vi "Example.vi"() -> ()   [LabVIEW 2014, in "TE Cooler.lvlib"]
uses:
  TE Cooler.lvlib
  <userlib>/_Session Fwk/Session - Root.lvclass
  reusable/Session APIs/File Access/Config Data/Config Data.lvclass
  reusable/Session APIs/File Access/Config Data/Config Session.ctl
  reusable/Session APIs/Session Log/System Log.lvclass
  TE Cooler.lvclass
  Data/TECData.lvclass
panel:
  out "error out":errorcluster
  out "Power":sgl
  in  "STOP":bool
  out "Input 1":sgl(graph)
  out "Input 2":sgl(graph)
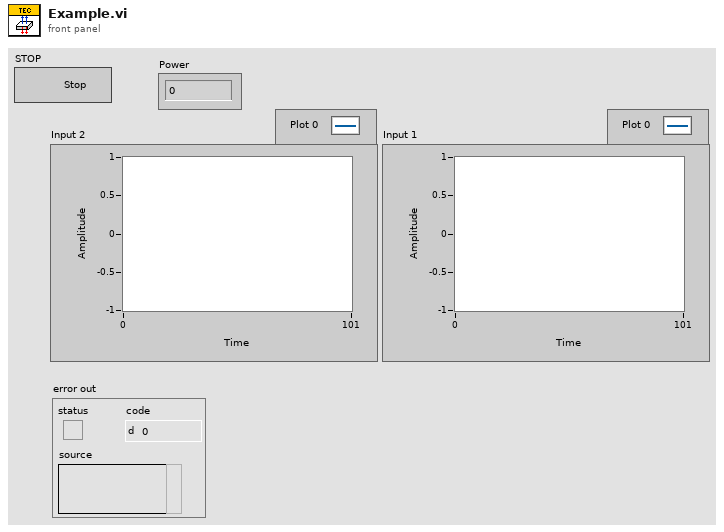
[diagram p1: front panel]
types:
  T1 = typedef "Config Data.lvclass/Config Session.ctl" = refnum<data-value>
  T2 = typedef "Session - Root.lvclass/Session Handle.ctl" = refnum<data-value>
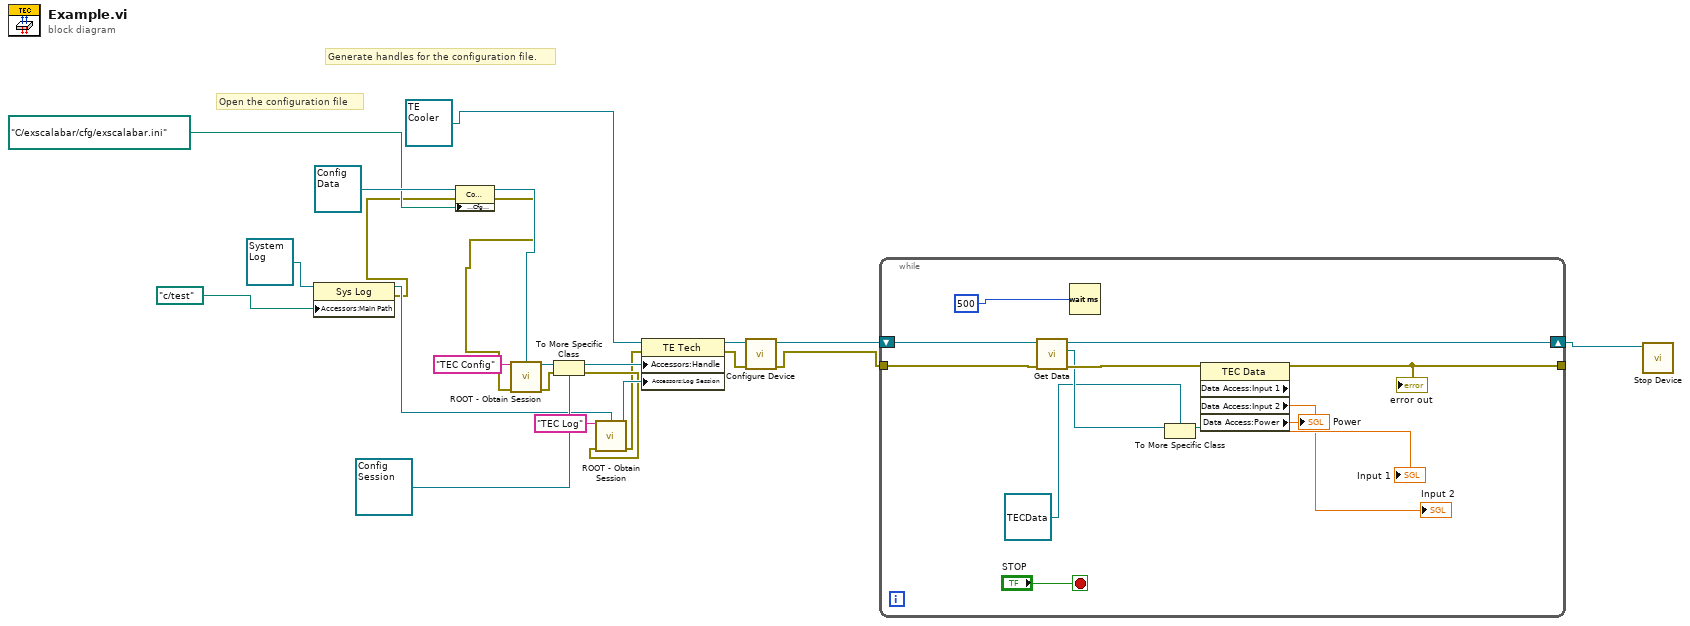
[diagram p0: block diagram]
diagram:
  # "Open the configuration file"
  # "Generate handles for the configuration file."
  n1 = property class="Sys Log"(reference=refnum<class "System Log.lvclass"> refnum ("Sys Log"), "Accessors:Main Path"=path "c:/test" ("Main Path")) -> (reference out=w15:refnum<class "System Log.lvclass">, error out=w4:errorcluster)  [unwired: 1 in]
  n2 = property class="Config Data"(reference=refnum<class "Config Data.lvclass"> refnum ("Config Data"), error in=w4, "Accessors:Cfg Path"=path "C:/exscalabar/cfg/exscalabar.ini" ("Path")) -> (reference out=w19:refnum<class "Config Data.lvclass">, error out=w18:errorcluster)
  n3 = call <userlib>:"ROOT - Obtain Session.vi"("Session Name ()"="TEC Config", "OBJ - Session"=w19, "error in (no error)"=w18) -> ("Session Handle"=w12:T2, "error out"=w10:errorcluster)  [unwired: 10 in, 1 out]
  n4 = To More Specific Class(target class=T1 refnum ("Session Handle"), reference=w12, error in=w10) -> (specific class reference=w11:T1, error out=w3:errorcluster)
  n5 = call <userlib>:"ROOT - Obtain Session.vi"("Session Name ()"="TEC Log", "OBJ - Session"=w15, "error in (no error)"=w3) -> ("Session Handle"=w9:T2, "error out"=w2:errorcluster)  [unwired: 10 in, 1 out]
  n6 = property class="TE Tech"(reference=refnum<class "TE Cooler.lvclass"> refnum ("TE Cooler.lvlib:TE Cooler.lvclass"), error in=w2, "Accessors:Handle"=w11, "Accessors:Log Session"=w9) -> (reference out=w14:refnum<class "TE Cooler.lvclass">, error out=w13:errorcluster)
  n7 = call-dynamic "Configure Device.vi"("error in"=w13, "Device in"=w14) -> ("error out"=w22:errorcluster, "Device out"=w23:refnum<class "TE Cooler.lvclass">)  [unwired: 6 in, 2 out]
  n8 = while {
    tunnel: w22 -> [w34]
    tunnel: [w33] -> _
    shift-right: [w32] -> w6
    shift-left: w23 -> [w35]
    stop <- "STOP" stop-if-true
    n9 = call-dynamic "Get Data.vi"("error in"=w34, "TE Cooler in"=w35) -> ("error out"=w33:errorcluster, "Data Out"=w28:refnum<class "Data.lvclass">, "TE Cooler out"=w32:refnum<class "TE Cooler.lvclass">)  [unwired: 7 in]
    "error out" <- w33
    n10 = Wait (ms)(milliseconds to wait=500) -> ()  [unwired: 1 out]
    n11 = To More Specific Class(target class=refnum<class "TECData.lvclass"> refnum ("TE Cooler.lvlib:TEC Data"), reference=w28) -> (specific class reference=w31:refnum<class "TECData.lvclass">)  [unwired: 1 in, 1 out]
    n12 = property class="TEC Data"(reference=w31) -> ("Data Access:Input 1"=→"Input 1":sgl, "Data Access:Input 2"=→"Input 2":sgl, "Data Access:Power"=→"Power":sgl)  [unwired: 1 in, 2 out]
  }
  n13 = call-dynamic "Stop Device.vi"("TE Cooler in"=w6) -> ()  [unwired: 9 in, 2 out]
